vi "Test Devices with Wi-Fi.vi"(8 "error in (no error)":errorcluster, 11 "Hardware Abstraction App in":refnum<class "Hardware Abstraction App.lvclass">) -> (0 "error out":errorcluster, 3 "Hardware Abstraction App out":refnum<class "Hardware Abstraction App.lvclass">)   [LabVIEW 2020, in "Hardware Abstraction App.lvclass"]
uses:
  Hardware Abstraction App.lvclass
  Devices/Arduino/Arduino.lvclass
  ESP8266/ESP8266.lvclass
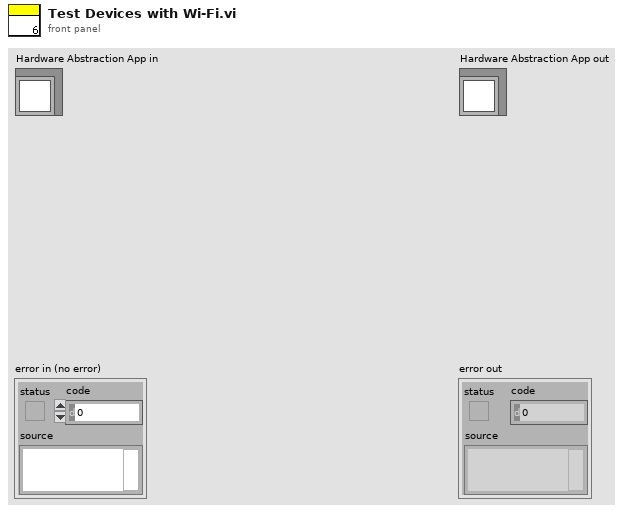
[diagram p1: front panel]
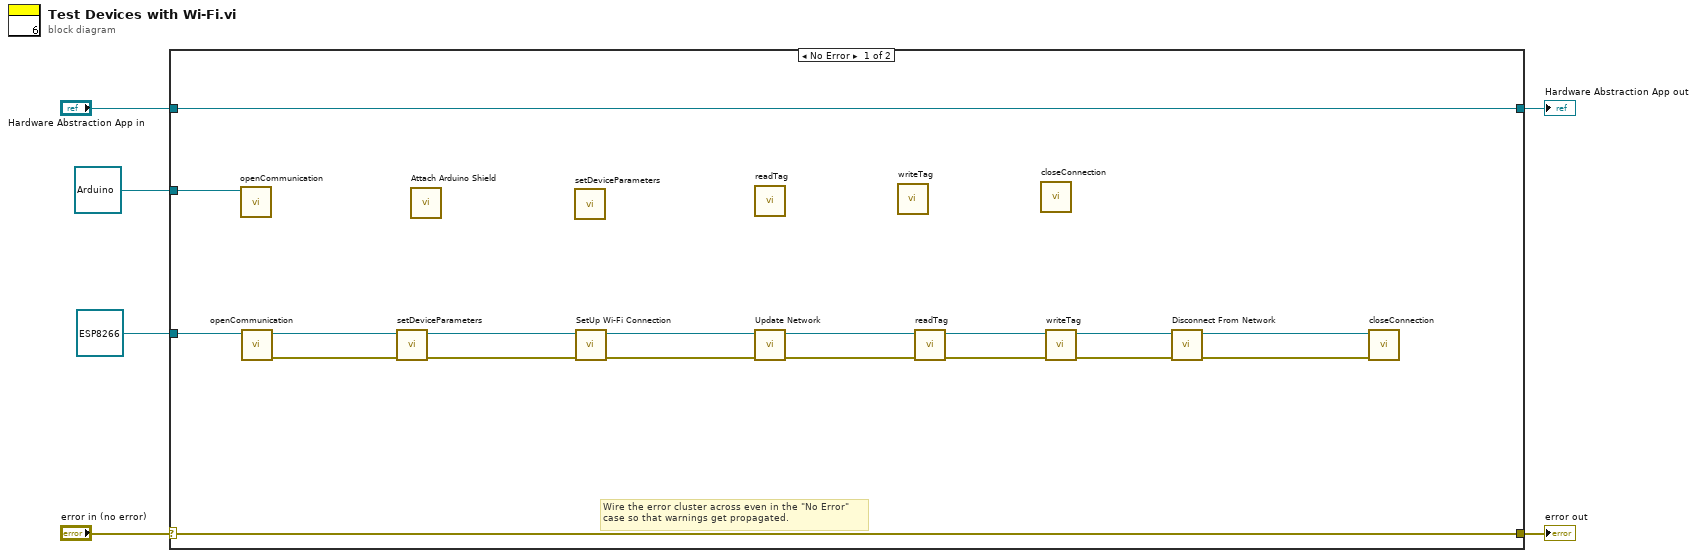
[diagram p0: block diagram]
diagram:
  n1 = case shown="No Error" "error in (no error)" {
    selector: "error in (no error)" -> [w23 w26]
    tunnel: [w23 w26] -> w5
    tunnel: [w24 w25] -> w3
    tunnel: "Hardware Abstraction App in" -> [w24 w25]
    tunnel: refnum<class "ESP8266.lvclass"> refnum ("ESP8266.lvclass") -> [w8 _]
    tunnel: refnum<class "Arduino.lvclass"> refnum ("Arduino.lvclass") -> [w7 _]
    frame No Error {
      # "Wire the error cluster across even in the \"No Error\"\ncase so that warnings get propagated."
      n2 = call-dynamic "openCommunication.vi"("Arduino in"=w7) -> ()  [unwired: 9 in, 2 out]
      n3 = call-dynamic "openCommunication.vi"("ESP8266 in"=w8) -> ("error out"=w21:errorcluster, "ESP8266 out"=w22:refnum<class "ESP8266.lvclass">)  [unwired: 9 in]
      n4 = call-dynamic "setDeviceParameters.vi"("error in (no error)"=w21, "ESP8266 in"=w22) -> ("error out"=w19:errorcluster, "ESP8266 out"=w20:refnum<class "ESP8266.lvclass">)  [unwired: 8 in]
      n5 = call "Attach Arduino Shield.vi"() -> ()  [unwired: 10 in, 2 out]
      n6 = call-dynamic "setDeviceParameters.vi"() -> ()  [unwired: 10 in, 2 out]
      n7 = call-dynamic "SetUp Wi-Fi Connection.vi"("error in (no error)"=w19, "ESP8266 in"=w20) -> ("error out"=w17:errorcluster, "ESP8266 out"=w18:refnum<class "ESP8266.lvclass">)  [unwired: 8 in]
      n8 = call-dynamic "readTag.vi"() -> ()  [unwired: 10 in, 2 out]
      n9 = call-dynamic "Update Network.vi"("error in (no error)"=w17, "ESP8266 in"=w18) -> ("error out"=w15:errorcluster, "ESP8266 out"=w16:refnum<class "ESP8266.lvclass">)  [unwired: 8 in]
      n10 = call-dynamic "writeTag.vi"() -> ()  [unwired: 10 in, 2 out]
      n11 = call-dynamic "readTag.vi"("error in (no error)"=w15, "ESP8266 in"=w16) -> ("error out"=w13:errorcluster, "ESP8266 out"=w14:refnum<class "ESP8266.lvclass">)  [unwired: 8 in]
      n12 = call-dynamic "closeConnection.vi"() -> ()  [unwired: 10 in, 2 out]
      n13 = call-dynamic "writeTag.vi"("error in (no error)"=w13, "ESP8266 in"=w14) -> ("error out"=w11:errorcluster, "ESP8266 out"=w12:refnum<class "ESP8266.lvclass">)  [unwired: 8 in]
      n14 = call-dynamic "Disconnect From Network.vi"("error in (no error)"=w11, "ESP8266 in"=w12) -> ("error out"=w9:errorcluster, "ESP8266 out"=w10:refnum<class "ESP8266.lvclass">)  [unwired: 8 in]
      n15 = call-dynamic "closeConnection.vi"("error in (no error)"=w9, "ESP8266 in"=w10) -> ()  [unwired: 8 in, 2 out]
    }
    frame Error {
    }
  }
  "error out" <- w5
  "Hardware Abstraction App out" <- w3
